vi "_VISA Read.vi"(8 "error in (no error)":errorcluster, 10 "Byte Count":u32=1024, 11 "VISA resource name":refnum<visa-resource-name>) -> (0 "error out":errorcluster, 2 "Response":string, 3 "VISA resource name out":refnum<visa-resource-name>)   [LabVIEW 2015, in "SRS SR400.lvlib"]
uses:
  SRS SR400.lvlib
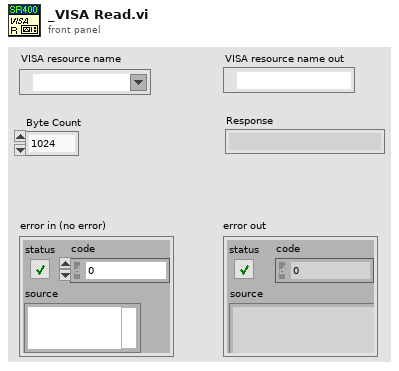
[diagram p1: front panel]
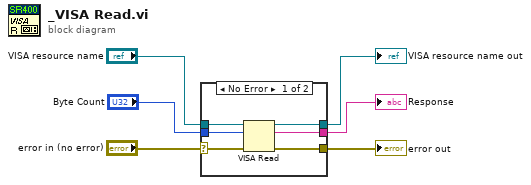
[diagram p0: block diagram]
diagram:
  n1 = case shown="No Error" "error in (no error)" {
    selector: "error in (no error)" -> [w7 w13]
    tunnel: [w12 w14] -> w6
    tunnel: [w11 w13] -> w5
    tunnel: [w10 _] -> w4
    tunnel: "Byte Count" -> [w9 _]
    tunnel: "VISA resource name" -> [w8 w14]
    frame No Error {
      n2 = VISA Read(VISA resource name=w8, byte count=w9, error in (no error)=w7) -> (VISA resource name out=w12:refnum<visa-resource-name>, read buffer=w10:string, error out=w11:errorcluster)  [unwired: 1 out]
    }
    frame Error {
    }
  }
  "VISA resource name out" <- w6
  "error out" <- w5
  "Response" <- w4
